vi "Read Measured value k1.vi"(8 "error in (no error)":errorcluster, 9 "Control system address":u8=208 format="%x", 10 "Component address":u8=16 format="%x", 11 "ELAN master in":refnum<class "ELAN Master.lvclass">) -> (0 "error out":errorcluster, 1 "channel state":T1, 2 "Value":T2 {"Value"."Value" format="%#_6f"}, 3 "ELAN master out":refnum<class "ELAN Master.lvclass">)   [LabVIEW 2021, in "ELAN Master.lvclass"]
doc: "Reads values from contiguous holding registers. The maximum number of holding registers this VI can read is 125."
uses:
  ELAN Master.lvclass
  Data Model/ELAN Data Model/Type Definitions/Value full.ctl
  Data Unit/ELAN PC Data Unit/Elan units.ctl
  Data Unit/ELAN PC Data Unit/Elan measured variable.ctl
  Data Unit/ELAN PC Data Unit/Elan channel state.ctl
  Data Unit/ELAN PC Data Unit/ELAN PDU.lvclass/ELAN PDU.ctl
  ELAN Master.lvclass/ELAN Master.ctl
  Transmission Data Unit/ELAN/ELAN Data Unit.lvclass/ELAN Data Unit.ctl
  Transmission Data Unit/ELAN/Write ADU Packet.vi
  Transmission Data Unit/ELAN/Read ADU Packet.vi
  Transmission Data Unit/ELAN/Write ACK Packet.vi
  Data Unit/ELAN PC Data Unit/Flatten PDU.vi
  Modbus_v121c/Network Interface/Serial Interface/Serial Shared Components/Serial Write.vi
  Transmission Data Unit/ELAN/Calculate CRC.vi
  Data Unit/ELAN PC Data Unit/Unflatten to PDU.vi
  Transmission Data Unit/ELAN/Check For Messages.vi
  <vilib>/Utility/error.llb/Error Cluster From Error Code.vi
  Data Unit/ELAN PC Data Unit/ELAN PDU.lvclass
  Data Model/ELAN Data Model/ELAN Data Model.lvclass
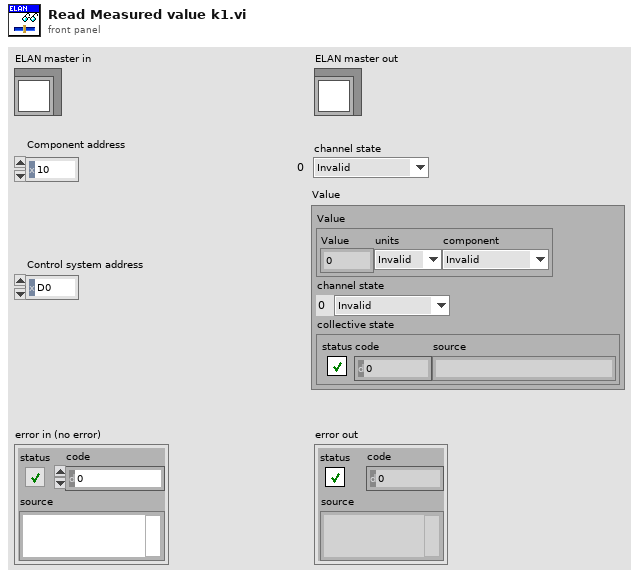
[diagram p1: front panel]
types:
  T1 = typedef "ELAN PDU.lvclass/Elan channel state.ctl" = enum16{"Invalid", "Warm-up", "Pause", "Standby", "Measure", "Zero calibration", "Adjust component slope", "Not yet defined1", "Adjust curve dip", "Adjust linearization sensitivity", "Adjust temperature compensation", "Adjust pressure compensation", "Adjust linearization zero", "Not yet defined2", "Autocal", "Adjust phase", "Zero calibration of O2 sensor", "Synchronous zero calibration", "Purging for synchronous zero calibration", "Adjust analog output", "Adjust analog input", "Autocal check"}
  T2 = typedef "ELAN Data Model.lvclass/Value full.ctl" = cluster{"Value":cluster{"Value":sgl, "units":T3, "component":T4}, "channel state":T1, "collective state":errorcluster}
  T3 = typedef "ELAN PDU.lvclass/Elan units.ctl" = enum16{"Invalid", "no dimension", "ppm", "ppb", "vpm", "ppm C1", "ppm C3", "ppm C6", "mg C/m3", "mg/m3", "%", "% vol", "% of measuring range", "% saturation", "%/°C", "%/K", "% weight", "mV/pH", "mV/mbar", "nA/mbar", "S/m", "S/cm", "mS/m", "mS/cm", "ìS/m", "ìS/cm", "S", "min", "H", "Pa", "MA", "uV", "MV", "V", "mbar", "hPa", "Ml/min", "kOhm", "MOhm", "S1", "°C", "Hz", "pH", "ug/l", "mg/l", "l/min", "uA", "mg/dm3", "kPa", "kOhm*cm", "MOhm*cm", "°", "1/min", "1/m", "g/m3", "g/l", "% Vol C"}
  T4 = typedef "ELAN PDU.lvclass/Elan measured variable.ctl" = enum16{"Invalid", "no component", "CO", "CO2", "CH4 (Methan)", "C6H14 (Hexan)", "SO2", "NO", "NO2", "CHClF2 (R22)", "C3H8 (Propan)", "C4H10 (Butan)", "O2", "C5H12 (Pentan)", "CnHm (THC)", "P (process pressure)", "pH", "T (temperature)", "C2H4 (Ethen)", "C2H2 (Ethin)", "C3H6 (Propen)", "C4H6", "C4H8", "C2H6", "NH3 (Ammoniak)", "N2O", "C6H6 (Benzol)", "SF6", "CH3OH (Methanol)", "C2H5OH (Ethanol)", "CH2Cl2", "C2H4Cl2", "CH3Cl", "C2H4O", "H2O (water vapor)", "G/l (conductivity)", "C", "S", "N", "CF4", "COCl2 (phosgene)", "CHF3 (R23)", "C2F6 (R116)", "------ (self defined component)", "C2H3Cl", "H2 (Hydrogen)", "Ar", "He", "Cl2", "N2"}
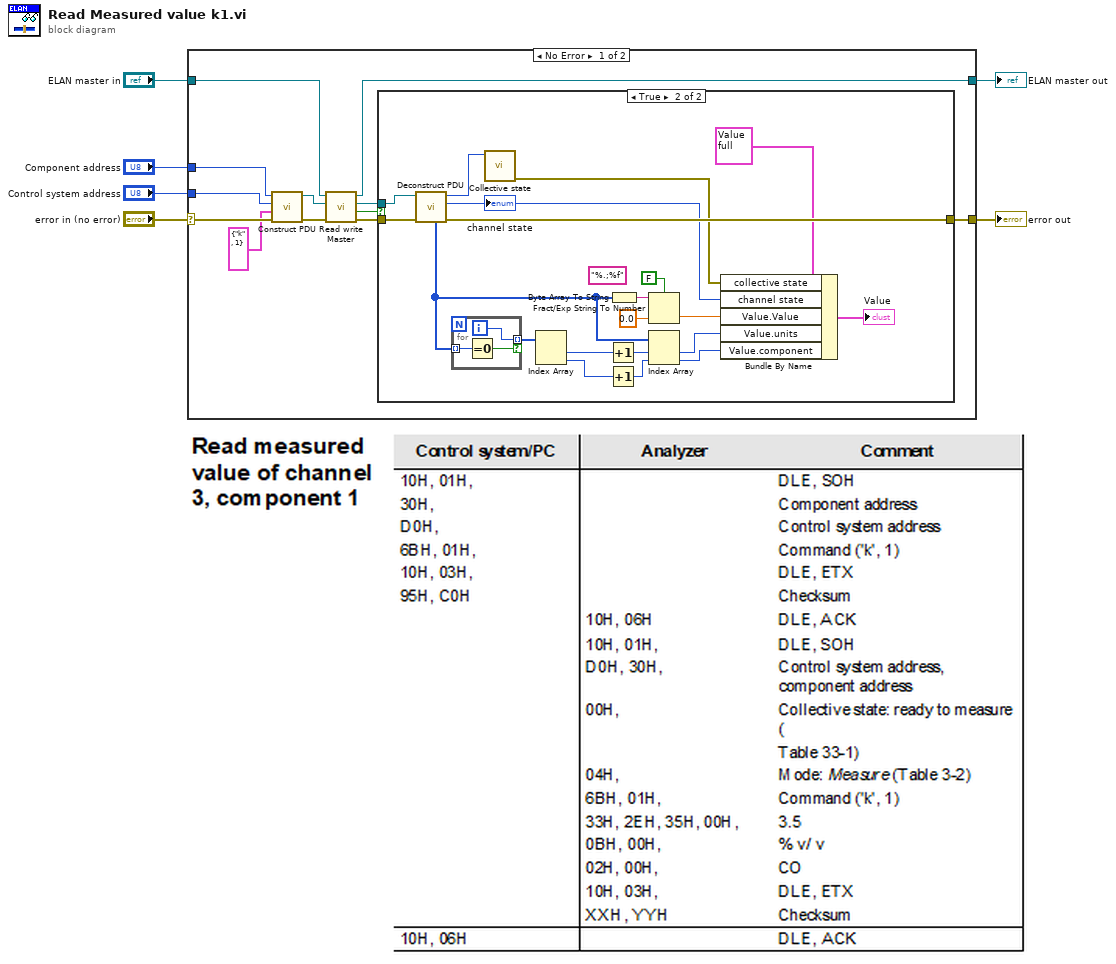
[diagram p0: block diagram]
diagram:
  n1 = case shown="No Error" "error in (no error)" {
    selector: "error in (no error)" -> [w11 w43]
    tunnel: "Control system address" -> [w7 _]
    tunnel: "Component address" -> [w8 _]
    tunnel: "ELAN master in" -> [w13 w44]
    tunnel: [w14 w44] -> w2
    tunnel: [w17 w43] -> w1
    frame No Error {
      n2 = call "Construct PDU.vi"("error in"=w11, "command"=cluster{"type":string, "number":u8} {"type"="k", "number"=1}, "source address"=w7, "target address"=w8) -> ("error out"=w10:errorcluster, "ELAN data unit out"=w12:refnum<class "ELAN PDU.lvclass">)  [unwired: 6 in]
      n3 = call "Read write Master.vi"("error in (no error)"=w10, "ELAN data unit in"=w12, "ELAN master in"=w13) -> ("error out"=w18:errorcluster, "PDU valid?"=w16:bool, "ELAN data unit out"=w15:refnum<class "ELAN PDU.lvclass">, "ELAN master out"=w14:refnum<class "ELAN Master.lvclass">)  [unwired: 5 in]
      n4 = case shown="True" w16 {
        tunnel: w18 -> [w19 w39]
        tunnel: [w19 w37] -> w17
        tunnel: w15 -> [_ w38]
        frame False {
        }
        frame True {
          (unwired) "%.;%f" ("format string")
          n5 = call "Deconstruct PDU.vi"("error in (no error)"=w39, "modbus data unit in"=w38) -> ("error out"=w37:errorcluster, "channel state"=w21:T1, "collective state"=w23:u8, "data"=w24:u8[])  [unwired: 3 in, 3 out]
          "channel state" <- w21
          n6 = for {
            tunnel: w24 -> [w42] mode=indexing
            tunnel: [w41] -> w33 mode=indexing if=w40
            i -> [w41]
            n7 = Equal To 0?(x=w42) -> (x = 0?=w40:bool)
          }
          n8 = call "Collective state.vi"("collective state"=w23) -> ("error out"=w20:errorcluster)  [unwired: 8 in, 2 out]
          n9 = Index Array(array=w33) -> (element #1=w26:i32, element #2=w25:i32)  [unwired: 2 in]
          n10 = Increment(x=w26) -> (x+1=w30:i32)
          n11 = Increment(x=w25) -> (x+1=w29:i32)
          n12 = Byte Array To String(unsigned byte array=w24) -> (string=w32:string)
          n13 = Fract/Exp String To Number(use system decimal point (T)=FALSE, string=w32, default (0 dbl)=sgl 0.0 ("default value 1")) -> (number=w31:sgl)  [unwired: 1 in, 1 out]
          n14 = Index Array(array=w24, index #1=w30, index #2=w29) -> (element #1=w28:u8, element #2=w27:u8)
          n15 = Bundle By Name(cluster=T2 {"Value"={"Value"=0.0, "units"=enum."Invalid", "component"=enum."Invalid"}, "channel state"=enum."Invalid", "collective state"={"status"=FALSE, "code"=0, "source"=""}} ("Value"), "collective state"=w20, "channel state"=w21, "Value.Value"=w31, "Value.units"=w28, "Value.component"=w27) -> (→"Value":T2)
        }
      }
    }
    frame Error {
    }
  }
  "ELAN master out" <- w2
  "error out" <- w1
